vi "Add Weighted Images (ARGB).vi"(5 "B":dbl=0.5, 6 "C (Default: 0)":dbl, 7 "A":dbl=0.5, 8 "error in (no error)":errorcluster, 9 "ARGB Image Destination in":T1, 10 "ARGB Image B in":T1, 11 "ARGB Image A in":T1) -> (0 "error out":errorcluster, 3 "ARGB Image Destination":T1)   [LabVIEW 2020, in "image.lvlib"]
doc: "Combine two images A and B scaled by their corresponding scaling factors - with the addition of an optional constant. Pixel values will saturate at their maximum values."
uses:
  image.lvlib
  ARGB Image.ctl
  000615f7-9334-4574-8f7b-324cbbba12df.vi
  <vilib>/Utility/error.llb/Error Cluster From Error Code.vi
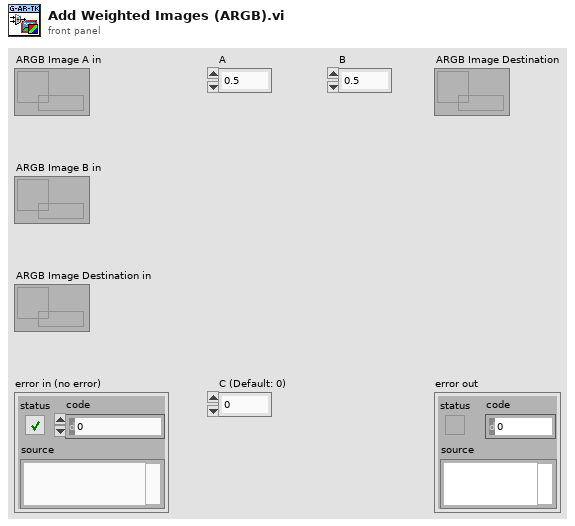
[diagram p1: front panel]
types:
  T1 = typedef "image.lvlib/ARGB Image.ctl" = refnum<data-value>
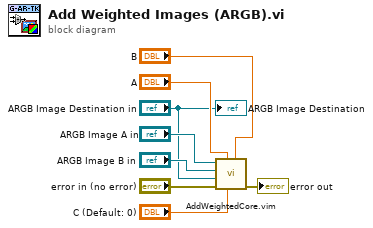
[diagram p0: block diagram]
diagram:
  n1 = call "AddWeightedCore.vim"("B"="B", "C"="C (Default: 0)", "A"="A", "error in (no error)"="error in (no error)", "Dst"="ARGB Image Destination in", "Image B"="ARGB Image B in", "Image A"="ARGB Image A in") -> ("error out"=→"error out":errorcluster)  [unwired: 4 in]
  "ARGB Image Destination" <- "ARGB Image Destination in"
